vi "RetriggeredAdvancedSequence.vi"() -> ()   [LabVIEW 2023]
doc: "Overview: This example demonstrates how to make sweep times faster by using LCR Advanced Sequence functions to change the frequency in a sequence. During the sequence, the channel steps through the predetermined set configurations (frequency in this example) without any interaction with the host system. The advantage of sequencing is that changes from one step in the sequence to the next are deterministic.\nThe program will perform an AC Voltage frequency sweep from Start Frequency to End Frequency. The sweep frequencies are an exponential sequence and the length of each of the sweeps is equal to the value in the Number Of Steps control."
uses:
  <instrlib>/niDCPower/nidcpower.llb/niDCPower Source Mode.ctl
  <instrlib>/niDCPower/nidcpower.llb/niDCPower Sequence Attribute Type.ctl
  <instrlib>/niDCPower/nidcpower.llb/niDCPower Wait For Event - Event.ctl
  <instrlib>/niDCPower/nidcpower.llb/niDCPower Send Software Edge Trigger - Signal.ctl
  <instrlib>/niDCPower/nidcpower.llb/niDCPower Configure Software Edge Sequence Advance Trigger With Channels.vi
  <instrlib>/niDCPower/nidcpower.llb/niDCPower Create Advanced Sequence Step With Channels.vi
panel:
  in  "Trigger":bool=TRUE
  in  "Stop Button":bool
  in  "Cable Length":i32(ring)=1122 items=["0m"=1121, "NI Standard 0.5m"=1153, "NI Standard 1m"=1122, "NI Standard 2m"=1123, "NI Standard 4m"=1124, "NI Standard Triaxial 1m"=1139, "NI Standard Triaxial 2m"=1140, "NI Standard Triaxial 4m"=1141, "Custom (Onboard Storage)"=1125, "Custom (As Configured)"=1126]
  in  "LCR Short Compensation Enabled":bool
  in  "LCR Open Compensation Enabled":bool
  in  "Impedance Range":dbl=100.0 format="%_6p"
  in  "LCR Custom Measurement Time Sec":dbl caption="LCR Custom \nMeasurement Time Sec" format="%_3p"
  in  "LCR Measurement Time":i32(ring)=1072 items=["Short"=1071, "Medium"=1072, "Long"=1073, "Custom"=1117]
  in  "LCR DC Bias Voltage":dbl caption="LCR DC Bias Voltage Level" format="%_3p"
  in  "LCR DC Bias Source":i32(ring)=1066 items=["Off"=1065, "Voltage"=1066, "Current"=1067]
  in  "Number of Steps":u32=100 caption="Number Of Steps"
  in  "End Frequency":dbl=500000.0 format="%#_3p"
  in  "Start Frequency":dbl=1000.0 format="%#_3p"
  in  "Voltage Amplitude RMS":dbl=0.7 format="%_6p"
  out "Impendance vs Frequency":T1(graph) caption="Impedance vs Frequency"
  in  "Channel Name":string="0"
  in  "Resource Name":refnum<k15>="Dev1"
  # "Overview: This example demonstrates how to make sweep times faster by using LCR Advanced Sequence functions to change the frequency in a sequence. During the sequence, the channel steps through the predetermined set configurations (frequency in this example) without any interaction with the host system. The advantage of sequencing is that changes from one step in the sequence to the next are deterministic. The program will perform an AC Voltage frequency sweep from Start Frequency to End Frequency. The sweep frequencies are an exponential sequence and the length of each of the sweeps is equal to the value in the Number Of Steps control. \n\nThe Cable Length option of \"Custom (As Configured)\" is not supported in this example. Search ni.com for information about NI power supplies/SMUs and the NI-DCPower API.\n\nRequirements: NI-DCPower\nInstructions:\n1. Select the appropriate instrument in the Resource Name control.\n2. Configure the parameters of the sweeps.\n3. Configure the Cable Length to match your cabling setup.\n4. Run the VI."
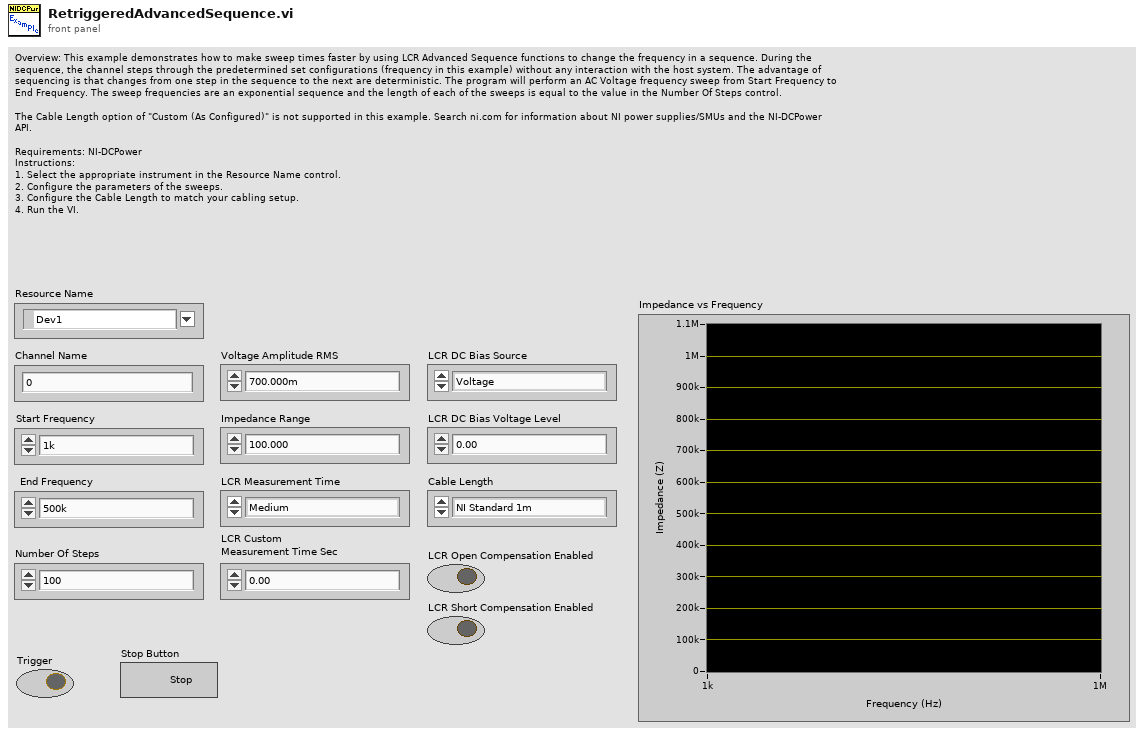
[diagram p1: front panel]
types:
  T1 = cluster{"voltage measurements":dbl[], "current measurements":dbl[]}
  T2 = typedef "niDCPower Sequence Attribute Type.ctl" = i32
  T3 = typedef "niDCPower Source Mode.ctl" = i32
  T4 = typedef "niDCPower Wait For Event - Event.ctl" = i32
  T5 = typedef "niDCPower LCR Measurement.ctl" = cluster{"V DC":dbl, "I DC":dbl, "stimulus frequency":dbl, "AC voltage":cdb, "AC current":cdb, "Z":cdb, "Z magnitude":dbl, "Z theta":dbl, "Y":cdb, "Y magnitude":dbl, "Y theta":dbl, "Ls":dbl, "Cs":dbl, "Rs":dbl, "Lp":dbl, "Cp":dbl, "Rp":dbl, "D":dbl, "Q":dbl, "measurement mode":u16, "DC in compliance":bool, "Pad 0":u8, "AC in compliance":bool, "Pad 1":u8, "unbalanced":bool, "Pad 2":u8, "Reserved 1":dbl, "Reserved 2":dbl, "Reserved 3":dbl, "Reserved 4":dbl, "Reserved 5":dbl, "Reserved 6":dbl, "Reserved 7":dbl}
  T6 = typedef "niDCPower Send Software Edge Trigger - Signal.ctl" = i32
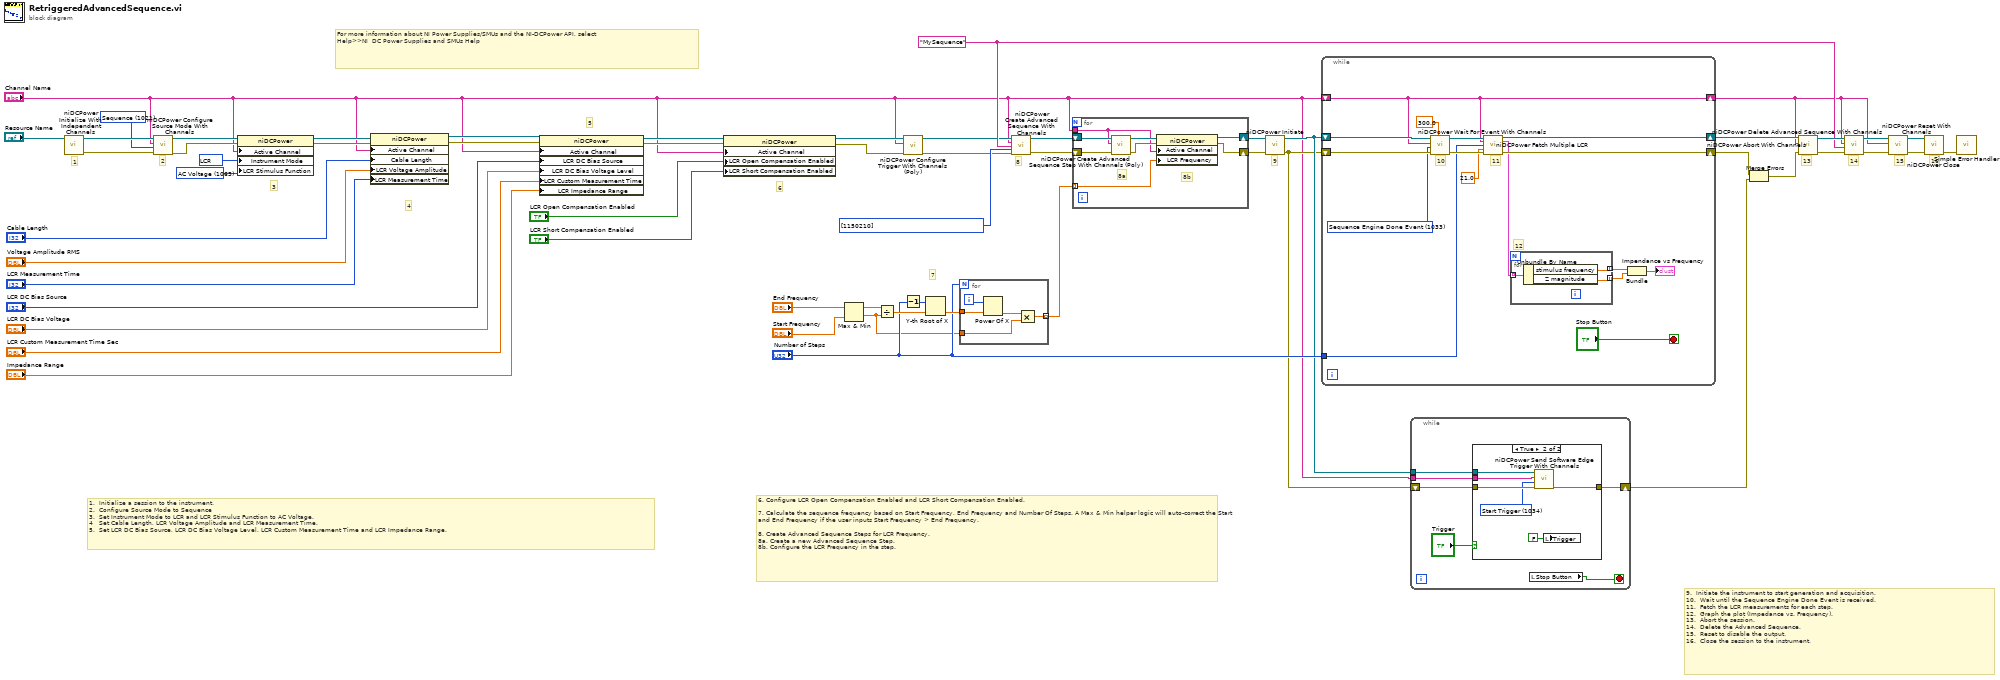
[diagram p0: block diagram]
diagram:
  w13 = T2[] [1150210] items=["Source -> Output Function"=1150008, "Source -> Output Enabled"=1250006, "Source -> Output Resistance"=1150061, "Source -> Transient Response"=1150062, "Source -> Custom Transient Response -> Voltage Gain Bandwidth"=1150067, "Source -> Custom Transient Response -> Voltage Compensation Frequency"=1150068, "Source -> Custom Transient Response -> Voltage Pole-Zero Ratio"=1150069, "Source -> Custom Transient Response -> Current Gain Bandwidth"=1150070, "Source -> Custom Transient Response -> Current Compensation Frequency"=1150071, "Source -> Custom Transient Response -> Current Pole-Zero Ratio"=1150072, "Source -> DC Voltage -> Voltage Level"=1250001, "Source -> DC Voltage -> Voltage Level Range"=1150005, "Source -> DC Voltage -> Current Limit"=1250005, "Source -> DC Voltage -> Current Limit High"=1150187, "Source -> DC Voltage -> Current Limit Low"=1150188, "Source -> DC Voltage -> Current Limit Range"=1150004, "Source -> DC Current -> Current Level"=1150009, "Source -> DC Current -> Current Level Range"=1150011, "Source -> DC Current -> Voltage Limit"=1150010, "Source -> DC Current -> Voltage Limit High"=1150185, "Source -> DC Current -> Voltage Limit Low"=1150186, "Source -> DC Current -> Voltage Limit Range"=1150012, "Source -> DC Current -> Current Level Slew Rate -> Rising"=1150343, "Source -> DC Current -> Current Level Slew Rate -> Falling"=1150344, "Source -> Pulse Voltage -> Pulse Voltage Level"=1150080, "Source -> Pulse Voltage -> Pulse Bias Voltage Level"=1150082, "Source -> Pulse Voltage -> Pulse Voltage Level Range"=1150084, "Source -> Pulse Voltage -> Pulse Current Limit"=1150081, "Source -> Pulse Voltage -> Pulse Current Limit High"=1150193, "Source -> Pulse Voltage -> Pulse Current Limit Low"=1150194, "Source -> Pulse Voltage -> Pulse Bias Current Limit"=1150083, "Source -> Pulse Voltage -> Pulse Bias Current Limit High"=1150195, "Source -> Pulse Voltage -> Pulse Bias Current Limit Low"=1150196, "Source -> Pulse Voltage -> Pulse Current Limit Range"=1150085, "Source -> Pulse Current -> Pulse Current Level"=1150086, "Source -> Pulse Current -> Pulse Bias Current Level"=1150088, "Source -> Pulse Current -> Pulse Current Level Range"=1150090, "Source -> Pulse Current -> Pulse Voltage Limit"=1150087, "Source -> Pulse Current -> Pulse Voltage Limit High"=1150189, "Source -> Pulse Current -> Pulse Voltage Limit Low"=1150190, "Source -> Pulse Current -> Pulse Bias Voltage Limit"=1150089, "Source -> Pulse Current -> Pulse Bias Voltage Limit High"=1150191, "Source -> Pulse Current -> Pulse Bias Voltage Limit Low"=1150192, "Source -> Pulse Current -> Pulse Voltage Limit Range"=1150091, "Source -> Advanced -> Source Delay"=1150051, "Source -> Advanced -> Pulse Bias Delay"=1150092, "Source -> Advanced -> Pulse On Time"=1150093, "Source -> Advanced -> Pulse Off Time"=1150094, "Source -> Advanced -> OVP Enabled"=1250002, "Source -> Advanced -> OVP Limit"=1250003, "Source -> Advanced -> Compliance Limit Symmetry"=1150184, "Source -> Advanced -> Sequence Step Delta Time"=1150198, "Source -> Advanced -> Conduction Voltage -> Mode"=1150350, "Source -> Advanced -> Conduction Voltage -> On Threshold"=1150351, "Source -> Advanced -> Conduction Voltage -> Off Threshold"=1150352, "Measurement -> Sense"=1150013, "Measurement -> Aperture Time"=1150058, "Measurement -> Measure Record Length"=1150063, "Measurement -> Advanced -> DC Noise Rejection"=1150066, "Measurement -> Autorange"=1150244, "Measurement -> Advanced -> Autorange Behavior"=1150245, "Measurement -> Advanced -> Autorange Aperture Time Mode"=1150246, "Measurement -> Advanced -> Autorange Minimum Aperture Time"=1150247, "Measurement -> Advanced -> Autorange Minimum Aperture Time Units"=1150248, "Measurement -> Advanced -> Autorange Minimum Current Range"=1150255, "Measurement -> Advanced -> Autorange Minimum Voltage Range"=1150256, "Measurement -> Advanced -> Autorange Threshold Mode"=1150257, "Measurement -> Advanced -> Autorange Maximum Delay After Range Change"=1150322, "LCR -> Instrument Mode"=1150208, "LCR -> Source Delay Mode"=1150315, "LCR -> Measurement Time"=1150218, "LCR -> Custom Measurement Time"=1150258, "LCR -> AC Stimulus -> Function"=1150209, "LCR -> AC Stimulus -> Frequency"=1150210, "LCR -> AC Stimulus -> Voltage Amplitude"=1150211, "LCR -> AC Stimulus -> Current Amplitude"=1150212, "LCR -> AC Stimulus -> Advanced -> Voltage Range"=1150265, "LCR -> AC Stimulus -> Advanced -> Current Range"=1150267, "LCR -> AC Stimulus -> Advanced -> Source Aperture Time"=1150349, "LCR -> DC Bias -> Source"=1150213, "LCR -> DC Bias -> Voltage Level"=1150214, "LCR -> DC Bias -> Current Level"=1150215, "LCR -> DC Bias -> Advanced -> Voltage Range"=1150266, "LCR -> DC Bias -> Advanced -> Current Range"=1150274, "LCR -> DC Bias -> Advanced -> Transient Response"=1150347, "LCR -> Compensation -> Open -> Enabled"=1150220, "LCR -> Compensation -> Open -> Conductance"=1150261, "LCR -> Compensation -> Open -> Susceptance"=1150262, "LCR -> Compensation -> Short -> Enabled"=1150221, "LCR -> Compensation -> Short -> Resistance"=1150263, "LCR -> Compensation -> Short -> Reactance"=1150264, "LCR -> Compensation -> Load -> Enabled"=1150222, "LCR -> Compensation -> Load -> Measured Resistance"=1150268, "LCR -> Compensation -> Load -> Measured Reactance"=1150269, "LCR -> Compensation -> Load -> Actual Resistance"=1150270, "LCR -> Compensation -> Load -> Actual Reactance"=1150271, "LCR -> Impedance Range -> Impedance Range"=1150217, "LCR -> Impedance Range -> Impedance Autorange"=1150216, "LCR -> Impedance Range -> Advanced -> Impedance Range Source"=1150321, "LCR -> Impedance Range -> Advanced -> Load Resistance"=1150318, "LCR -> Impedance Range -> Advanced -> Load Inductance"=1150319, "LCR -> Impedance Range -> Advanced -> Load Capacitance"=1150320] ("advanced sequence properties")
  w33 = 1063 items=["AC Voltage"=1063, "AC Current"=1064] ("LCR:AC Stimulus:Function")
  w34 = 1062 items=["SMU PS"=1061, "LCR"=1062] ("LCR:Instrument Mode")
  w42 = "MySequence" ("sequence name")
  w52 = T3 1021 items=["Single Point"=1020, "Sequence"=1021] ("source mode")
  # "1"
  # "5"
  # "7"
  # "6. Configure LCR Open Compensation Enabled and LCR Short Compensation Enabled.\n\n7. Calculate the sequence frequency based on Start Frequency, End Frequency and Number Of Steps. A Max & Min helper logic will auto-correct the Start and End Frequency if the user inputs Start Frequency > End Frequency.\n\n8. Create Advanced Sequence Steps for LCR Frequency.\n8a. Create a new Advanced Sequence Step.\n8b. Configure the LCR Frequency in the step."
  # "6"
  # "4"
  # "3"
  # "8"
  # "13"
  # "14"
  # "9.  Initiate the instrument to start generation and acquisition.\n10.  Wait until the Sequence Engine Done Event is received.\n11.  Fetch the LCR measurements for each step.\n12.  Graph the plot (Impedance vs. Frequency).\n13.  Abort the session.\n14.  Delete the Advanced Sequence.\n15.  Reset to disable the output.\n16.  Close the session to the instrument."
  # "For more information about NI Power Supplies/SMUs and the NI-DCPower API, select\nHelp>>NI  DC Power Supplies and SMUs Help"
  # "16"
  # "9"
  # "2"
  # "1.  Initialize a session to the instrument.\n2.  Configure Source Mode to Sequence \n3.  Set Instrument Mode to LCR and LCR Stimulus Function to AC Voltage.\n4   Set Cable Length, LCR Voltage Amplitude and LCR Measurement Time. \n5.  Set LCR DC Bias Source, LCR DC Bias Voltage Level, LCR Custom Measurement Time and LCR Impedance Range."
  # "15"
  n1 = call <instrlib>:"niDCPower Initialize With Independent Channels.vi"("resource name"="Resource Name") -> ("error out"=w54:errorcluster, "instrument handle out"=w53:refnum<k15>)  [unwired: 9 in]
  n2 = call <instrlib>:"niDCPower Configure Source Mode With Channels.vi"("error in (no error)"=w54, "source mode"=w52, "channel name"="Channel Name", "instrument handle"=w53) -> ("error out"=w45:errorcluster, "instrument handle out"=w46:refnum<k15>)  [unwired: 6 in]
  n3 = property class="niDCPower"(reference=w46, error in=w45, "Active Channel"="Channel Name", "Instrument Mode"=w34, "LCR Stimulus Function"=w33) -> (reference out=w24:refnum<k15>, error out=w23:errorcluster)
  n4 = property class="niDCPower"(reference=w24, error in=w23, "Active Channel"="Channel Name", "Cable Length"="Cable Length", "LCR Voltage Amplitude"="Voltage Amplitude RMS", "LCR Measurement Time"="LCR Measurement Time") -> (reference out=w22:refnum<k15>, error out=w21:errorcluster)
  n5 = property class="niDCPower"(reference=w22, error in=w21, "Active Channel"="Channel Name", "LCR DC Bias Source"="LCR DC Bias Source", "LCR DC Bias Voltage Level"="LCR DC Bias Voltage", "LCR Custom Measurement Time"="LCR Custom Measurement Time Sec", "LCR Impedance Range"="Impedance Range") -> (reference out=w28:refnum<k15>, error out=w27:errorcluster)
  n6 = property class="niDCPower"(reference=w28, error in=w27, "Active Channel"="Channel Name", "LCR Open Compensation Enabled"="LCR Open Compensation Enabled", "LCR Short Compensation Enabled"="LCR Short Compensation Enabled") -> (reference out=w9:refnum<k15>, error out=w11:errorcluster)
  n7 = Max & Min(x="End Frequency", y="Start Frequency") -> (max(x,y)=w29:dbl, min(x,y)=w30:dbl)
  n8 = Divide(x=w29, y=w30) -> (x/y=w38:dbl)
  n9 = call-poly <instrlib>:"niDCPower Configure Trigger With Channels (Poly).vi"("error in (no error)"=w11, "channel name"="Channel Name", "instrument handle"=w9) -> ("error out"=w10:errorcluster, "instrument handle out"=w8:refnum<k15>)  [unwired: 7 in]
  n10 = Decrement(x="Number of Steps") -> (x-1=w39:u32)
  n11 = Y-th Root of X(1:w38, 2:w39) -> (0:w37:dbl)
  n12 = for {
    N: "Number of Steps" -> [_]
    tunnel: w30 -> [w59]
    tunnel: w37 -> [w62]
    tunnel: [w58] -> w36 mode=indexing
    i -> [w61]
    n13 = Power Of X(1:w62, 2:w61) -> (0:w60:dbl)
    n14 = Multiply(x=w60, y=w59) -> (x*y=w58:dbl)
  }
  n15 = call <instrlib>:"niDCPower Create Advanced Sequence With Channels.vi"("instrument handle"=w8, "channel name"="Channel Name", "sequence name"=w42, "advanced sequence properties"=w13, "error in (no error)"=w10) -> ("instrument handle out"=w44:refnum<k15>, "error out"=w43:errorcluster)  [unwired: 9 in]
  n16 = for {
    shift-right: [w67] -> w40
    shift-left: w43 -> [w70]
    tunnel: w36 -> [w64] mode=indexing
    tunnel: "Channel Name" -> [w63]
    shift-right: [w65] -> w41
    shift-left: w44 -> [w69]
    # "8b"
    # "8a"
    n17 = call-poly <instrlib>:"niDCPower Create Advanced Sequence Step With Channels (Poly).vi"("error in (no error)"=w70, "channel name"=w63, "instrument handle"=w69) -> ("error out"=w66:errorcluster, "instrument handle out"=w68:refnum<k15>)  [unwired: 7 in]
    n18 = property class="niDCPower"(reference=w68, error in=w66, "Active Channel"=w63, "LCR Frequency"=w64) -> (reference out=w65:refnum<k15>, error out=w67:errorcluster)
  }
  n19 = call <instrlib>:"niDCPower Initiate.vi"("error in (no error)"=w40, "instrument handle"=w41) -> ("error out"=w6:errorcluster, "instrument handle out"=w7:refnum<k15>)  [unwired: 2 in, 6 out]
  n20 = while {
    tunnel: "Number of Steps" -> [w80]
    shift-right: [w81] -> w48
    shift-left: w7 -> [w86]
    shift-right: [w82] -> w4
    shift-left: w6 -> [w84]
    shift-right: [w71] -> w1
    shift-left: "Channel Name" -> [w71]
    stop <- "Stop Button" stop-if-true
    w72 = T4 1033 items=["Source Complete Event"=1030, "Measure Complete Event"=1031, "Sequence Iteration Complete Event"=1032, "Sequence Engine Done Event"=1033] ("event")
    # "11"
    # "10"
    # "12"
    n21 = call <instrlib>:"niDCPower Wait For Event With Channels.vi"("timeout (10.0)"=300.0, "error in (no error)"=w84, "event"=w72, "channel name"=w71, "instrument handle"=w86) -> ("error out"=w83:errorcluster, "instrument handle out"=w85:refnum<k15>)  [unwired: 5 in]
    n22 = call <instrlib>:"niDCPower Fetch Multiple LCR.vi"("instrument handle"=w85, "channel name"=w71, "count (1)"=w80, "timeout (1.0)"=21.0, "error in (no error)"=w83) -> ("instrument handle out"=w81:refnum<k15>, "measurements"=w79:T5[], "error out"=w82:errorcluster)  [unwired: 7 in, 1 out]
    n23 = for {
      tunnel: w79 -> [w89] mode=indexing
      tunnel: [w88] -> w78 mode=indexing
      tunnel: [w87] -> w77 mode=indexing
      n24 = Unbundle By Name(w89) -> ("stimulus frequency"=w88:dbl, "Z magnitude"=w87:dbl)
    }
    n25 = Bundle(w78, w77) -> (→"Impendance vs Frequency":cluster{dbl[], dbl[]})  [unwired: 1 out]
  }
  n26 = while {
    tunnel: w7 -> [w93]
    tunnel: "Channel Name" -> [w91]
    shift-right: [w90] -> w2
    shift-left: w6 -> [w92]
    stop <- w94 stop-if-true
    n27 = case shown="True" "Trigger" {
      tunnel: w93 -> [_ w102]
      tunnel: w92 -> [w96 w101]
      tunnel: w91 -> [_ w100]
      tunnel: [w96 w98] -> w90
      frame False {
      }
      frame True {
        w99 = T6 1034 items=["Start Trigger"=1034, "Source Trigger"=1035, "Measure Trigger"=1036, "Sequence Advance Trigger"=1037, "Pulse Trigger"=1053, "Shutdown Trigger"=1118] ("signal")
        n28 = call <instrlib>:"niDCPower Send Software Edge Trigger With Channels.vi"("error in (no error)"=w101, "signal"=w99, "channel name"=w100, "instrument handle"=w102) -> ("error out"=w98:errorcluster)  [unwired: 6 in, 1 out]
        n29 = local write "Trigger"(FALSE ("Trigger")) -> ()
      }
    }
    n30 = local read "Stop Button"() -> (w94:bool)
  }
  n31 = Merge Errors(w4, w2) -> (w3:errorcluster)
  n32 = call <instrlib>:"niDCPower Abort With Channels.vi"("error in (no error)"=w3, "channel name"=w1, "instrument handle"=w48) -> ("error out"=w49:errorcluster, "instrument handle out"=w47:refnum<k15>)  [unwired: 7 in]
  n33 = call <instrlib>:"niDCPower Delete Advanced Sequence With Channels.vi"("error in (no error)"=w49, "sequence name"=w42, "channel name"=w1, "instrument handle"=w47) -> ("error out"=w51:errorcluster, "instrument handle out"=w50:refnum<k15>)  [unwired: 6 in]
  n34 = call <instrlib>:"niDCPower Reset With Channels.vi"("error in (no error)"=w51, "channel name"=w1, "instrument handle"=w50) -> ("error out"=w56:errorcluster, "instrument handle out"=w57:refnum<k15>)  [unwired: 7 in]
  n35 = call <instrlib>:"niDCPower Close.vi"("error in (no error)"=w56, "instrument handle"=w57) -> ("error out"=w55:errorcluster)  [unwired: 9 out]
  n36 = call <vilib>:"Simple Error Handler.vi"("error in (no error)"=w55) -> ()  [unwired: 1 in, 8 out]
